vi "MH_GetFeatures.vi"(8 "error in (no error)":errorcluster, 11 "devidx":i32) -> (0 "error out":errorcluster, 2 "features":i32, 3 "return type":i32)   [LabVIEW 2019]
uses:
  <userlib>/MultiHarp150/MH_DllPath_global.vi
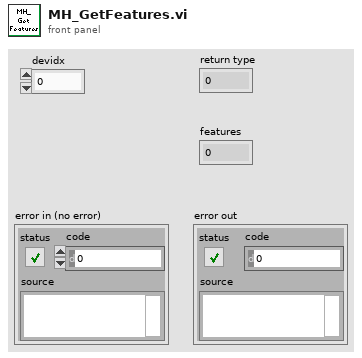
[diagram p1: front panel]
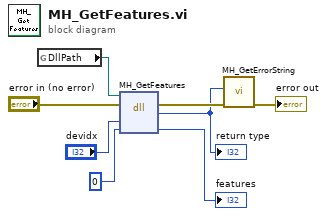
[diagram p0: block diagram]
diagram:
  n1 = global read "MH_DllPath_global.vi" "DllPath"() -> (w7:path)
  n2 = dll-call lib="MHLib64.dll" fn="MH_GetFeatures"(path in=w7, error in="error in (no error)", "devidx"="devidx", "features"=0 ("ctcstatus")) -> (error out=w5:errorcluster, "return type"=w4:i32, "features"=→"features":i32)  [unwired: 2 in, 1 out]
  "return type" <- w4
  n3 = call <userlib>:"MH_GetErrorString.vi"("error in (no error)"=w5, "code"=w4) -> ("error out"=→"error out":errorcluster)  [unwired: 7 in, 2 out]
